vi "Autonomous Independent.vi"() -> ()   [LabVIEW 2016]
doc: "This VI is called when autonomous begins, and will automatically be terminated when autonomous ends. You can carry out timed or sensor driven robot movement independently without needing to return to the caller."
uses:
  <vilib>/Rock Robotics/WPI/RobotDrive/WPI_RobotDriveMecanumDrive_Cartesian.vi
  <vilib>/Rock Robotics/Network Tables/NT Write Numeric Array.vi
  Global 4.vi
  <vilib>/Rock Robotics/Network Tables/NT Read String.vi
panel:
  out "Team Red?":bool
  out "Team Blue?":bool
  out "Current Movement, for debugging":T1 {"Z Joystick Value" scale=-1.0..1.0; "Y Joystick Value" scale=1.0..-1.0; "X Joystick Value" scale=-1.0..1.0}
  in  "Array of robot movements":T2(array[cluster])=[{"X Joystick Value"=-0.010101010101010017, "Y Joystick Value"=0.0, "Z Joystick Value"=0.4574773480918073, "Delay (sec)"=0.0, "Movement Name"=""}, {"X Joystick Value"=0.050505050505050594, "Y Joystick Value"=0.0, "Z Joystick Value"=-0.25616029503917137, "Delay (sec)"=0.0, "Movement Name"=""}] {"Z Joystick Value" scale=-1.0..1.0; "Y Joystick Value" scale=1.0..-1.0; "X Joystick Value" scale=-1.0..1.0}
  # "Be sure to right-click and choose Data Operations>>Make Current Value default if you want to save the array values with the VI"
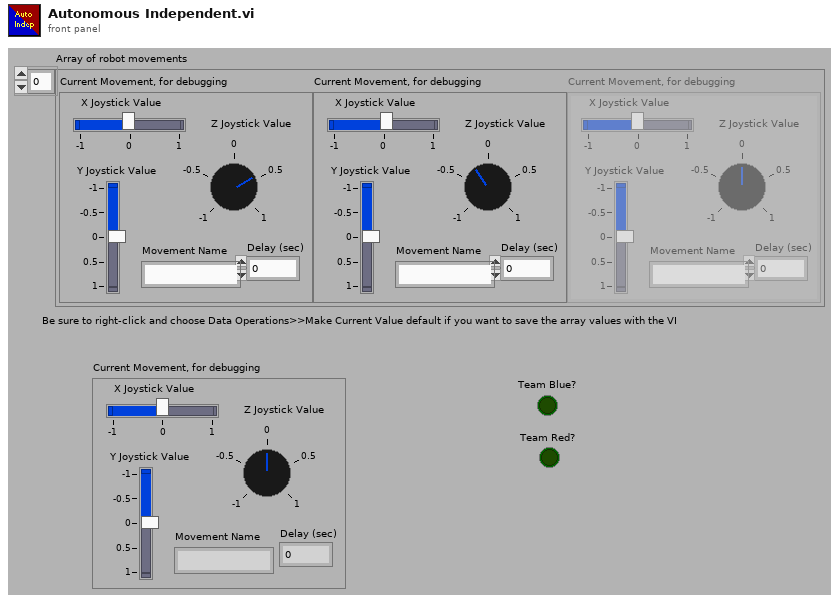
[diagram p1: front panel]
types:
  T1 = cluster{"X Joystick Value":dbl, "Y Joystick Value":dbl, "Z Joystick Value":dbl, "Delay (sec)":dbl, "Movement Name":string}
  T2 = cluster{"X Joystick Value":dbl, "Y Joystick Value":dbl, "Z Joystick Value":dbl, "Delay (sec)":dbl, "Movement Name":string}[]
  T3 = typedef "WPI_DriverStationAllianceInfo.ctl" = enum16{"Red", "Blue", "Invalid"}
  T4 = typedef "WPI_JoystickDevRef.ctl" = cluster{"Device":T5}
  T5 = typedef "WPI_JoystickDeviceEnum.ctl" = enum16{"USB 0", "USB 1", "USB 2", "USB 3", "USB 4", "USB 5"}
  T6 = cluster{"Boolean array[0]":bool, "Boolean array[1]":bool, "Boolean array[2]":bool, "Boolean array[3]":bool, "Boolean array[4]":bool, "Boolean array[5]":bool, "Boolean array[6]":bool, "Boolean array[7]":bool, "Boolean array[8]":bool}
  T7 = typedef "WPI_RobotDriveDevRef.ctl" = cluster{"DevStatus":errorcluster, "Motors[]":T8[], "Square Inputs":bool, "Max Output":dbl}
  T8 = typedef "WPI_MotorControlDeviceRef.ctl" = cluster{"DeviceStatus":errorcluster, "Type":T9, "PWM":cluster{"PWM Channel":T10, "DeadBand":T11}, "CAN":cluster{"Device Number":u8, "SetOutput VI Ref":variant, "GetOutput VI Ref":variant, "Enable VI Ref":variant, "Disable VI Ref":variant, "Data":variant}, "Invert":bool}
  T9 = typedef "WPI_MotorControlType.ctl" = enum16{"PWM", "CAN"}
  T10 = typedef "FPGA_DIOPWMChannel.ctl" = enum8{"PWM 0", "PWM 1", "PWM 2", "PWM 3", "PWM 4", "PWM 5", "PWM 6", "PWM 7", "PWM 8", "PWM 9", "PWM MXP 0", "PWM MXP 1", "PWM MXP 2", "PWM MXP 3", "PWM MXP 4", "PWM MXP 5", "PWM MXP 6", "PWM MXP 7", "PWM MXP 8", "PWM MXP 9", "Invalid"}
  T11 = typedef "WPI_PWMDeadband.ctl" = cluster{"Name":string, "maxPositivePwm":i32, "minPositivePwm":i32, "centerPwm":i32, "maxNegativePwm":i32, "minNegativePwm":i32, "angularRange":u16}
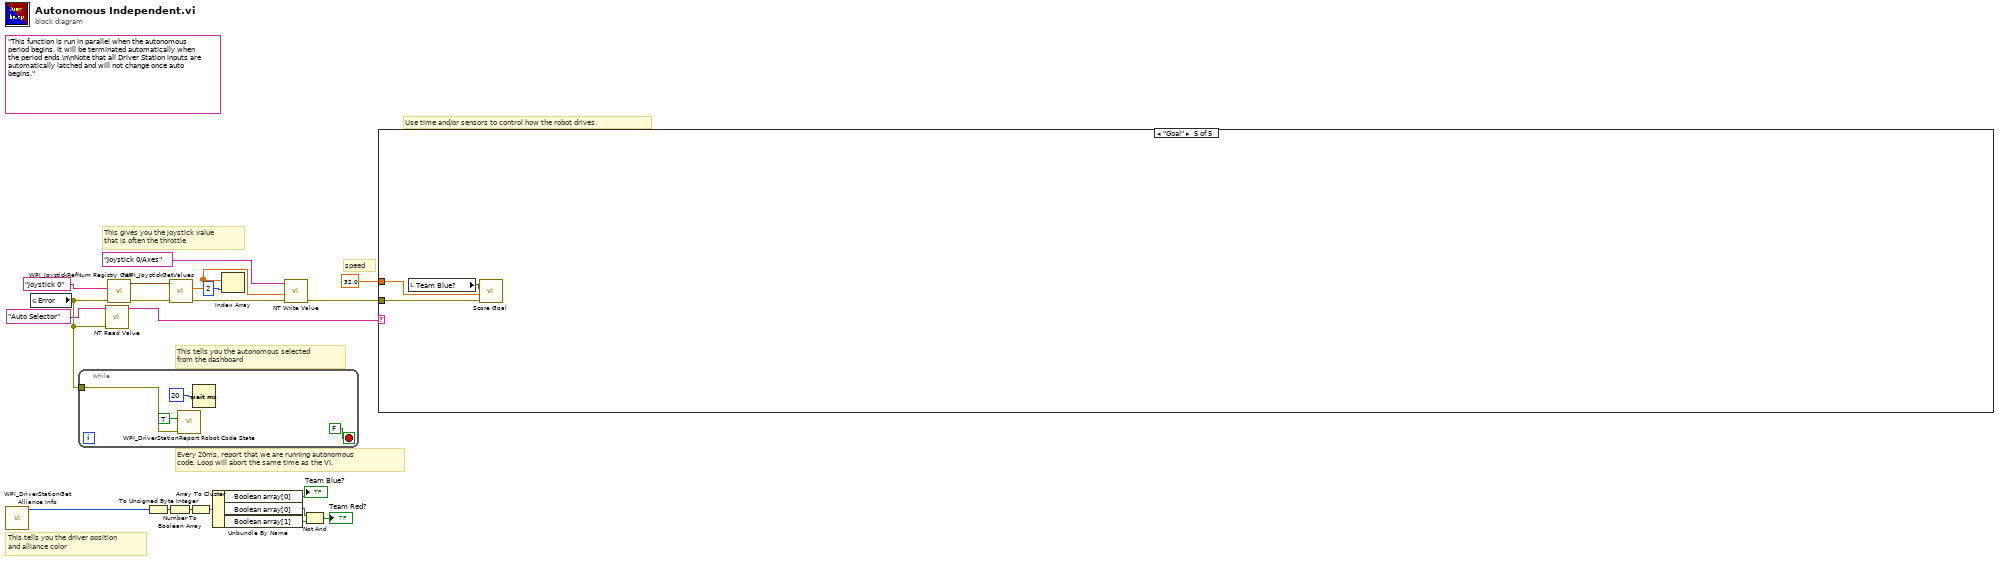
[diagram p0: block diagram]
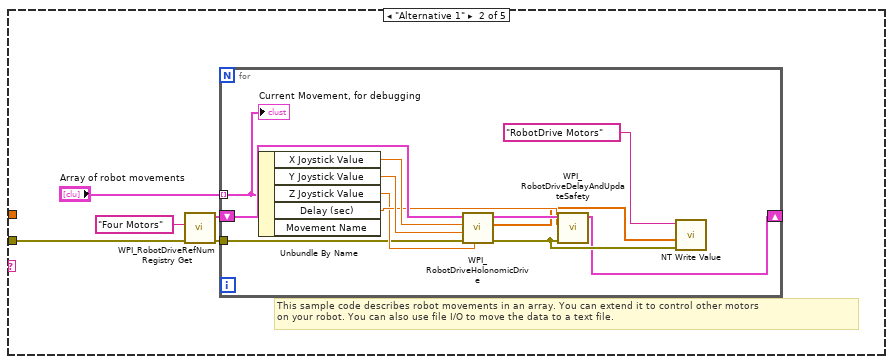
[diagram p3: hidden frame]
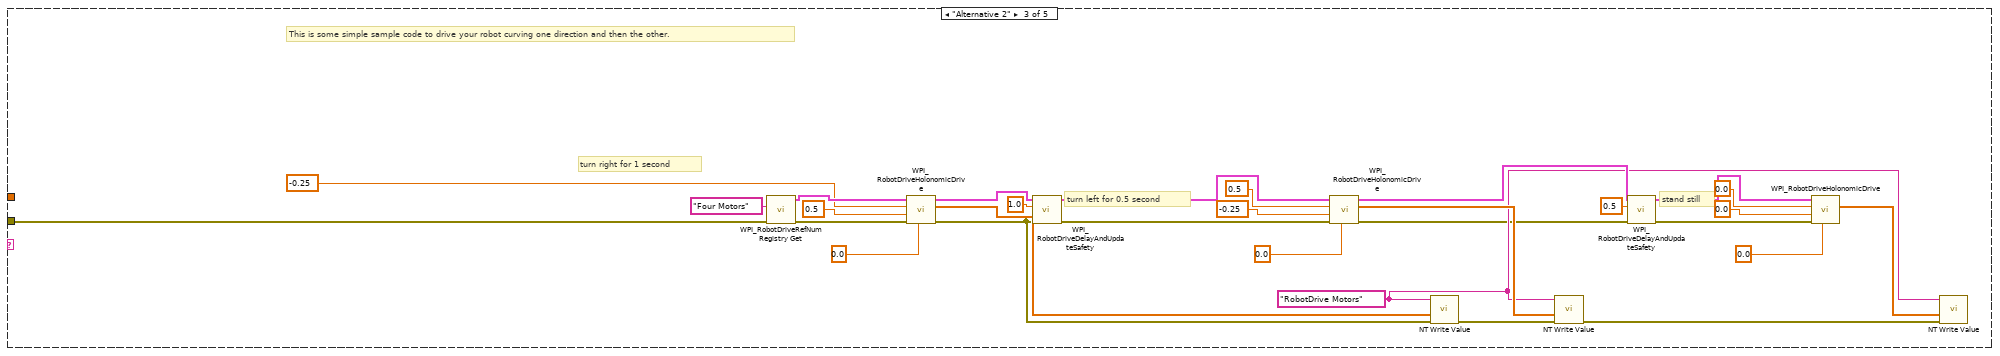
[diagram p4: hidden frame]
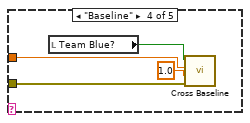
[diagram p5: hidden frame]
diagram:
  (unwired) "This function is run in parallel when the autonomous period begins. It will be terminated automatically when the period ends.\n\nNote that all Driver Station inputs are automatically latched and will not change once auto begins."
  # "speed"
  # "This tells you the autonomous selected\nfrom the dashboard"
  # "Every 20ms, report that we are running autonomous\ncode. Loop will abort the same time as the VI."
  # "This gives you the joystick value\nthat is often the throttle"
  # "Use time and/or sensors to control how the robot drives."
  # "This tells you the driver position\nand alliance color"
  n1 = call <vilib>:"WPI_DriverStationGet Alliance Info.vi"() -> ("Alliance"=w3:T3)  [unwired: 11 out]
  n2 = global read "Global 4.vi" "Error"() -> (w2:errorcluster)
  n3 = while {
    tunnel: w2 -> [w21]
    stop <- FALSE stop-if-true
    n4 = call <vilib>:"WPI_DriverStationReport Robot Code State.vi"("error in (no error)"=w21, "Autonomous"=TRUE) -> ()  [unwired: 9 in, 1 out]
    n5 = Wait (ms)(milliseconds to wait=u32 20) -> ()  [unwired: 1 out]
  }
  n6 = call-poly <vilib>:"NT Read Value.vi"("error in"=w2, "Name"="Auto Selector") -> ("String"=w16:string)  [unwired: 8 in, 1 out]
  n7 = call <vilib>:"WPI_JoystickRefNum Registry Get.vi"("error in (no error)"=w2, "refnum name"="Joystick 0") -> ("error out"=w13:errorcluster, "JoystickDevRef"=w19:T4)  [unwired: 8 out]
  n8 = To Unsigned Byte Integer(number=w3) -> (unsigned 8bit integer=w4:u8)
  n9 = Number To Boolean Array(number=w4) -> (Boolean array=w10:bool[])
  n10 = call <vilib>:"WPI_JoystickGetValues.vi"("error in (no error)"=w13, "JoystickDevRef"=w19) -> ("error out"=w12:errorcluster, "Axes"=w14:dbl[])  [unwired: 5 in, 3 out]
  n11 = Array To Cluster(array=w10) -> (cluster=w9:T6)
  n12 = Unbundle By Name(w9) -> ("Boolean array[0]"=→"Team Blue?":bool, "Boolean array[0]"=w7:bool, "Boolean array[1]"=w6:bool)
  n13 = Index Array(array=w14, index=2 ("milliseconds to wait")) -> ()  [unwired: 1 out]
  n14 = call-poly <vilib>:"NT Write Value.vi"("error in"=w12, "Numeric Array"=w14, "Name"="Joystick 0/Axes") -> ("error out"=w11:errorcluster)  [unwired: 8 in]
  n15 = Not And(1:w6, 2:w7) -> (0:→"Team Red?":bool)
  n16 = case shown="\"Goal\"" w16 {
    tunnel: w11 -> [_ w28 w42 w74 w76]
    tunnel: 32.0 -> [_ _ _ w71 w75]
    frame Default {
      # "You can put your main auto here, or you can right-click on the case and make any\nother frame be the default case."
      # "This is the frame that will execute if no selection is made, or if it is not recognized"
    }
    frame "Alternative 1" {
      # "This sample code describes robot movements in an array. You can extend it to control other motors\non your robot. You can also use file I/O to move the data to a text file."
      n17 = call <vilib>:"WPI_RobotDriveRefNum Registry Get.vi"("error in (no error)"=w28, "refnum name"="Four Motors") -> ("error out"=w26:errorcluster, "RobotDriveDevRef"=w27:T7)  [unwired: 8 out]
      n18 = for {
        shift-right: [w30] -> _
        shift-left: w27 -> [w40]
        tunnel: "Array of robot movements" -> [w36] mode=indexing
        tunnel: w26 -> [w31]
        n19 = Unbundle By Name(w36) -> ("X Joystick Value"=w39:dbl, "Y Joystick Value"=w38:dbl, "Z Joystick Value"=w35:dbl, "Delay (sec)"=w37:dbl)  [unwired: 1 out]
        n20 = call-poly <vilib>:"WPI_RobotDriveHolonomicDrive.vi"("Rotation"=w35, "error in (no error)"=w31, "Y"=w38, "X"=w39, "RobotDriveDevRef"=w40) -> ("error out"=w32:errorcluster, "Motor Values"=w33:dbl[], "RobotDriveDevRef"=w41:T7)  [unwired: 4 in]
        n21 = call <vilib>:"WPI_RobotDriveDelayAndUpdateSafety.vi"("error in (no error)"=w32, "Delay (s)"=w37, "RobotDriveDevRef"=w41) -> ("RobotDriveDevRef 2"=w30:T7)  [unwired: 7 in, 1 out]
        n22 = call-poly <vilib>:"NT Write Value.vi"("error in"=w32, "Numeric Array"=w33, "Name"="RobotDrive Motors") -> ()  [unwired: 8 in, 1 out]
        "Current Movement, for debugging" <- w36
      }
    }
    frame "Alternative 2" {
      w50 = "RobotDrive Motors" ("Name")
      # "This is some simple sample code to drive your robot curving one direction and then the other."
      # "stand still"
      # "turn left for 0.5 second"
      # "turn right for 1 second"
      n23 = call <vilib>:"WPI_RobotDriveRefNum Registry Get.vi"("error in (no error)"=w42, "refnum name"="Four Motors") -> ("error out"=w49:errorcluster, "RobotDriveDevRef"=w67:T7)  [unwired: 8 out]
      n24 = call-poly <vilib>:"WPI_RobotDriveHolonomicDrive.vi"("Rotation"=0.0, "error in (no error)"=w49, "Y"=0.5 ("X axis value"), "X"=-0.25 ("X axis value"), "RobotDriveDevRef"=w67) -> ("error out"=w45:errorcluster, "Motor Values"=w51:dbl[], "RobotDriveDevRef"=w60:T7)  [unwired: 4 in]
      n25 = call <vilib>:"WPI_RobotDriveDelayAndUpdateSafety.vi"("error in (no error)"=w45, "Delay (s)"=1.0, "RobotDriveDevRef"=w60) -> ("error out"=w48:errorcluster, "RobotDriveDevRef 2"=w61:T7)  [unwired: 7 in]
      n26 = call-poly <vilib>:"WPI_RobotDriveHolonomicDrive.vi"("Rotation"=0.0, "error in (no error)"=w48, "Y"=-0.25 ("X axis value"), "X"=0.5 ("X axis value"), "RobotDriveDevRef"=w61) -> ("error out"=w47:errorcluster, "Motor Values"=w52:dbl[], "RobotDriveDevRef"=w62:T7)  [unwired: 4 in]
      n27 = call-poly <vilib>:"NT Write Value.vi"("error in"=w45, "Numeric Array"=w51, "Name"=w50) -> ("error out"=w44:errorcluster)  [unwired: 8 in]
      n28 = call-poly <vilib>:"NT Write Value.vi"("error in"=w44, "Numeric Array"=w52, "Name"=w50) -> ("error out"=w43:errorcluster)  [unwired: 8 in]
      n29 = call <vilib>:"WPI_RobotDriveDelayAndUpdateSafety.vi"("error in (no error)"=w47, "Delay (s)"=0.5, "RobotDriveDevRef"=w62) -> ("error out"=w46:errorcluster, "RobotDriveDevRef 2"=w63:T7)  [unwired: 7 in]
      n30 = call-poly <vilib>:"WPI_RobotDriveHolonomicDrive.vi"("Rotation"=0.0 ("X axis value"), "error in (no error)"=w46, "Y"=0.0 ("X axis value"), "X"=0.0 ("X axis value"), "RobotDriveDevRef"=w63) -> ("Motor Values"=w53:dbl[])  [unwired: 4 in, 2 out]
      n31 = call-poly <vilib>:"NT Write Value.vi"("error in"=w43, "Numeric Array"=w53, "Name"=w50) -> ()  [unwired: 8 in, 1 out]
    }
    frame "Baseline" {
      n32 = local read "Team Blue?"() -> (w73:bool)
      n33 = call "Cross Baseline.vi"("error in (no error)"=w74, "Image Scale Factor"=sgl 1.0, "Speed (ft/s)"=w71, "Team Blue?"=w73) -> ()  [unwired: 7 in, 1 out]
    }
    frame "Goal" {
      n34 = local read "Team Blue?"() -> (w77:bool)
      n35 = call "Score Goal.vi"("error in (no error)"=w76, "Speed"=w75, "Team Blue?"=w77) -> ()  [unwired: 8 in, 1 out]
    }
  }
